vi "Setup_Onenote_Application.vi"(8 "error in (no error)":errorcluster, 11 "Array":string[](array[string])=["Asana_Authorization_Code.txt", "OneNote_Access_Token.txt", "OneNote_Refresh_Token.txt"]) -> (0 "error out":errorcluster, 3 "Paths":T1)   [LabVIEW 2016]
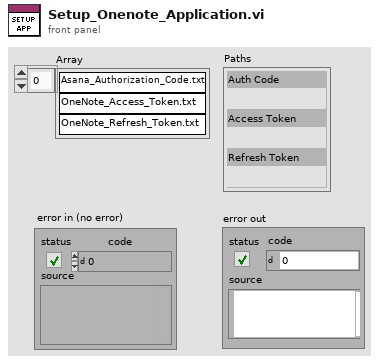
[diagram p1: front panel]
types:
  T1 = cluster{"Auth Code":path, "Access Token":path, "Refresh Token":path}
  T2 = enum16{"open", "replace", "create", "open or create", "replace or create", "replace or create with confirmation"}
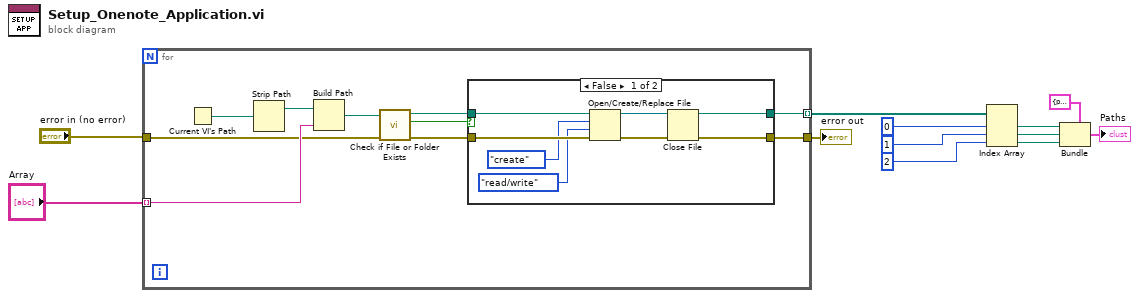
[diagram p0: block diagram]
diagram:
  n1 = for {
    tunnel: "Array" -> [w20] mode=indexing
    tunnel: [w17] -> w9 mode=indexing
    tunnel: [w15] -> w11
    tunnel: "error in (no error)" -> [w13]
    n2 = Current VI's Path() -> (path=w22:path)
    n3 = Strip Path(path=w22) -> (stripped path=w21:path)  [unwired: 1 out]
    n4 = Build Path(base path=w21, name or relative path=w20) -> (appended path=w19:path)
    n5 = call <vilib>:"Check if File or Folder Exists.vi"("error in (no error)"=w13, "path"=w19) -> ("error out"=w16:errorcluster, "file or folder exists?"=w14:bool, "dup path"=w18:path)  [unwired: 7 in]
    n6 = case shown="False" w14 {
      tunnel: w18 -> [w30 w32]
      tunnel: [w28 w32] -> w17
      tunnel: w16 -> [w27 w31]
      tunnel: [w23 w31] -> w15
      frame False {
        n7 = Open/Create/Replace File(file path (use dialog)=w30, error in=w27, operation (0:open)=T2."create", access (0:read/write)=enum16{"read/write", "read-only", "write-only"}."read/write") -> (refnum out=w29:refnum<file>, error out=w26:errorcluster)  [unwired: 2 in, 1 out]
        n8 = Close File(refnum=w29, error in=w26) -> (path=w28:path, error out=w23:errorcluster)
      }
      frame True {
      }
    }
  }
  "error out" <- w11
  n9 = Index Array(array=w9, index #1=0 ("index"), index #2=1 ("index"), index #3=2 ("index")) -> (element #1=w5:path, element #2=w4:path, element #3=w3:path)
  n10 = Bundle(cluster=T1 {"Auth Code"=path "", "Access Token"=path "", "Refresh Token"=path ""}, "Auth Code"=w5, "Access Token"=w4, "Refresh Token"=w3) -> (→"Paths":T1)
